vi "Semaphore Timed Wait (absolute seconds).vi"(8 "error in (no error)":errorcluster, 10 "absolute timeout (seconds)":dbl, 11 "Semaphore in":T1) -> (0 "error out":errorcluster, 2 "timed out?":bool, 3 "Semaphore out":T1)   [LabVIEW 2013, in "Linux RT IPC.POSIX Threads.lvlib" / "Semaphore.lvclass"]
doc: "Calls sem_timedwait() on the semaphore object encapsulated by Semaphore.\n\nThis VI attempts to decrement the value of the semaphore by 1 within a timeout period. If the semaphore can be decremented within the timeout period, this VI returns indicating it was successful. Otherwise, this VI returns indicating the semaphore was never set.\n\nTo provide a valid absolute timeout, query the Realtime clock for the current time and offset the time by the desired timeout duration.\n\nRefer to online POSIX documentation for more information."
uses:
  Semaphore.lvclass
  Controls/reference.ctl
  POSIX Thread Object/POSIX Thread Object.lvclass/POSIX Thread Object.ctl
  POSIX Thread Object/Private VIs/libpthread path.vi
  <vilib>/NI/NI Linux RT Utilities/VIs/Public/Convert Types/convert timespec 64 to timespec 32.vi
  POSIX Thread Object/Private VIs/get pthread error.vi
  <vilib>/NI/NI Linux RT Errno/VIs/Public/SubVIs/errno enum to number.vi
  <vilib>/NI/NI Linux RT Errno/VIs/Public/Get Errno Value for Calling Thread.vi
  POSIX Thread Object/POSIX Thread Object.lvclass
  <vilib>/NI/NI Linux RT Utilities/Linux RT Utilities.lvlib
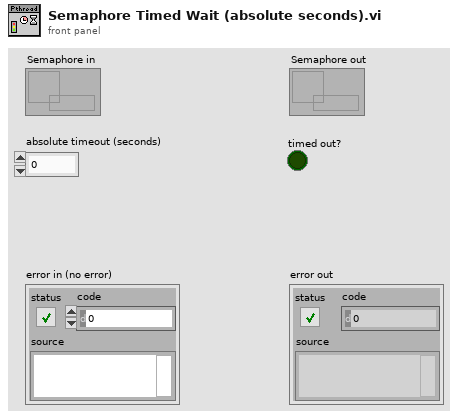
[diagram p1: front panel]
types:
  T1 = typedef "Linux RT IPC.POSIX Threads.lvlib/Semaphore.lvclass/reference.ctl" = refnum<data-value>
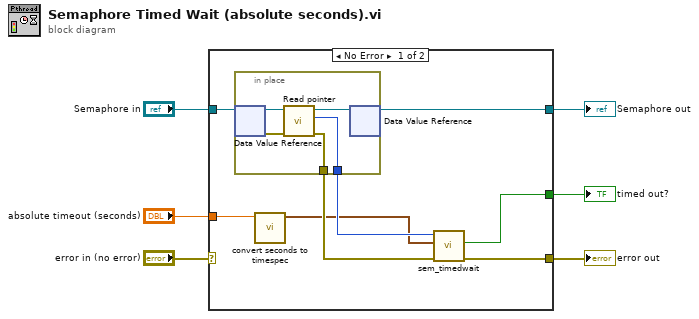
[diagram p0: block diagram]
diagram:
  n1 = case shown="No Error" "error in (no error)" {
    selector: "error in (no error)" -> [_ w20]
    tunnel: "Semaphore in" -> [w14 w21]
    tunnel: [w13 w21] -> w3
    tunnel: [w11 w20] -> w4
    tunnel: "absolute timeout (seconds)" -> [w8 _]
    tunnel: [w9 _] -> w1
    frame No Error {
      n2 = in-place {
        in-place-border: [w16] -> w12
        in-place-border: [w15] -> w10
        n3 = in-place-dvr #1(w14) -> (w19:refnum<class "Semaphore.lvclass">, w18:errorcluster)
        n4 = call "Read pointer.vi"("error in (no error)"=w18, "POSIX Thread Object in"=w19) -> ("error out"=w16:errorcluster, "pointer"=w15:u64, "POSIX Thread Object out"=w17:refnum<class "Semaphore.lvclass">)  [unwired: 7 in]
        n5 = in-place-dvr #1(w17) -> (w13:T1)  [unwired: 1 out]
      }
      n6 = call <vilib>:"convert seconds to timespec.vi"("seconds"=w8) -> ("timespec"=w7:cluster{"sec":u64, "nsec":u64})  [unwired: 10 in]
      n7 = call "sem_timedwait.vi"("error in (no error)"=w12, "absolute timeout"=w7, "sempahore ptr in"=w10) -> ("error out"=w11:errorcluster, "timed out?"=w9:bool)  [unwired: 6 in, 1 out]
    }
    frame Error {
    }
  }
  "error out" <- w4
  "Semaphore out" <- w3
  "timed out?" <- w1
